vi "数据处理整合 (子VI).vi"(11 "枚举":enum16{"实时数据排序", "小时数据排序"}(ring)) -> (3 "已排序的数组":string[](array[string]))   [LabVIEW 2016, in "数据传输系统-04.lvlib"]
uses:
  <userlib>/_OpenG.lib/array/array.llb/Remove Duplicates from 1D Array (String)__ogtk.vi
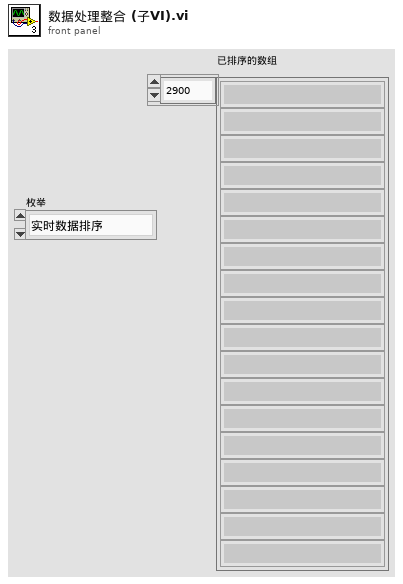
[diagram p1: front panel]
types:
  T1 = cluster{"PH":string[][], "CODCr":string[][], "氨氮":string[][], "CODMn":string[][], "总氮":string[][], "总磷":string[][], "电导率":string[][], "水温":string[][], "COD":string[][], "DO":string[][], "浊度":string[][], "叶绿素":string[][], "藻密度":string[][], "铜":string[][], "盐度":string[][], "水位":string[][], "流速":string[][], "方向":string[][], "瞬时流量":string[][], "累积流量":string[][], "正累积流量":string[][], "负累积流量":string[][], "亚硝酸盐":string[][], "硫化物":string[][], "ORP":string[][], "铅":string[][], "镉":string[][], "锌":string[][], "镍":string[][], "锰":string[][], "汞":string[][], "气温":string[][], "气压":string[][], "风速":string[][], "风向":string[][], "空气温度":string[][], "相对湿度":string[][], "分钟雨量":string[][], "小时雨量":string[][], "日雨量":string[][], "累积雨量":string[][], "盐度":string[][], "磷酸盐":string[][], "硝氮":string[][], "氟化物":string[][], "挥发酚":string[][], "氯化物":string[][], "蓝绿藻":string[][], "余氯":string[][], "综合生物毒性":string[][], "水深":string[][]}
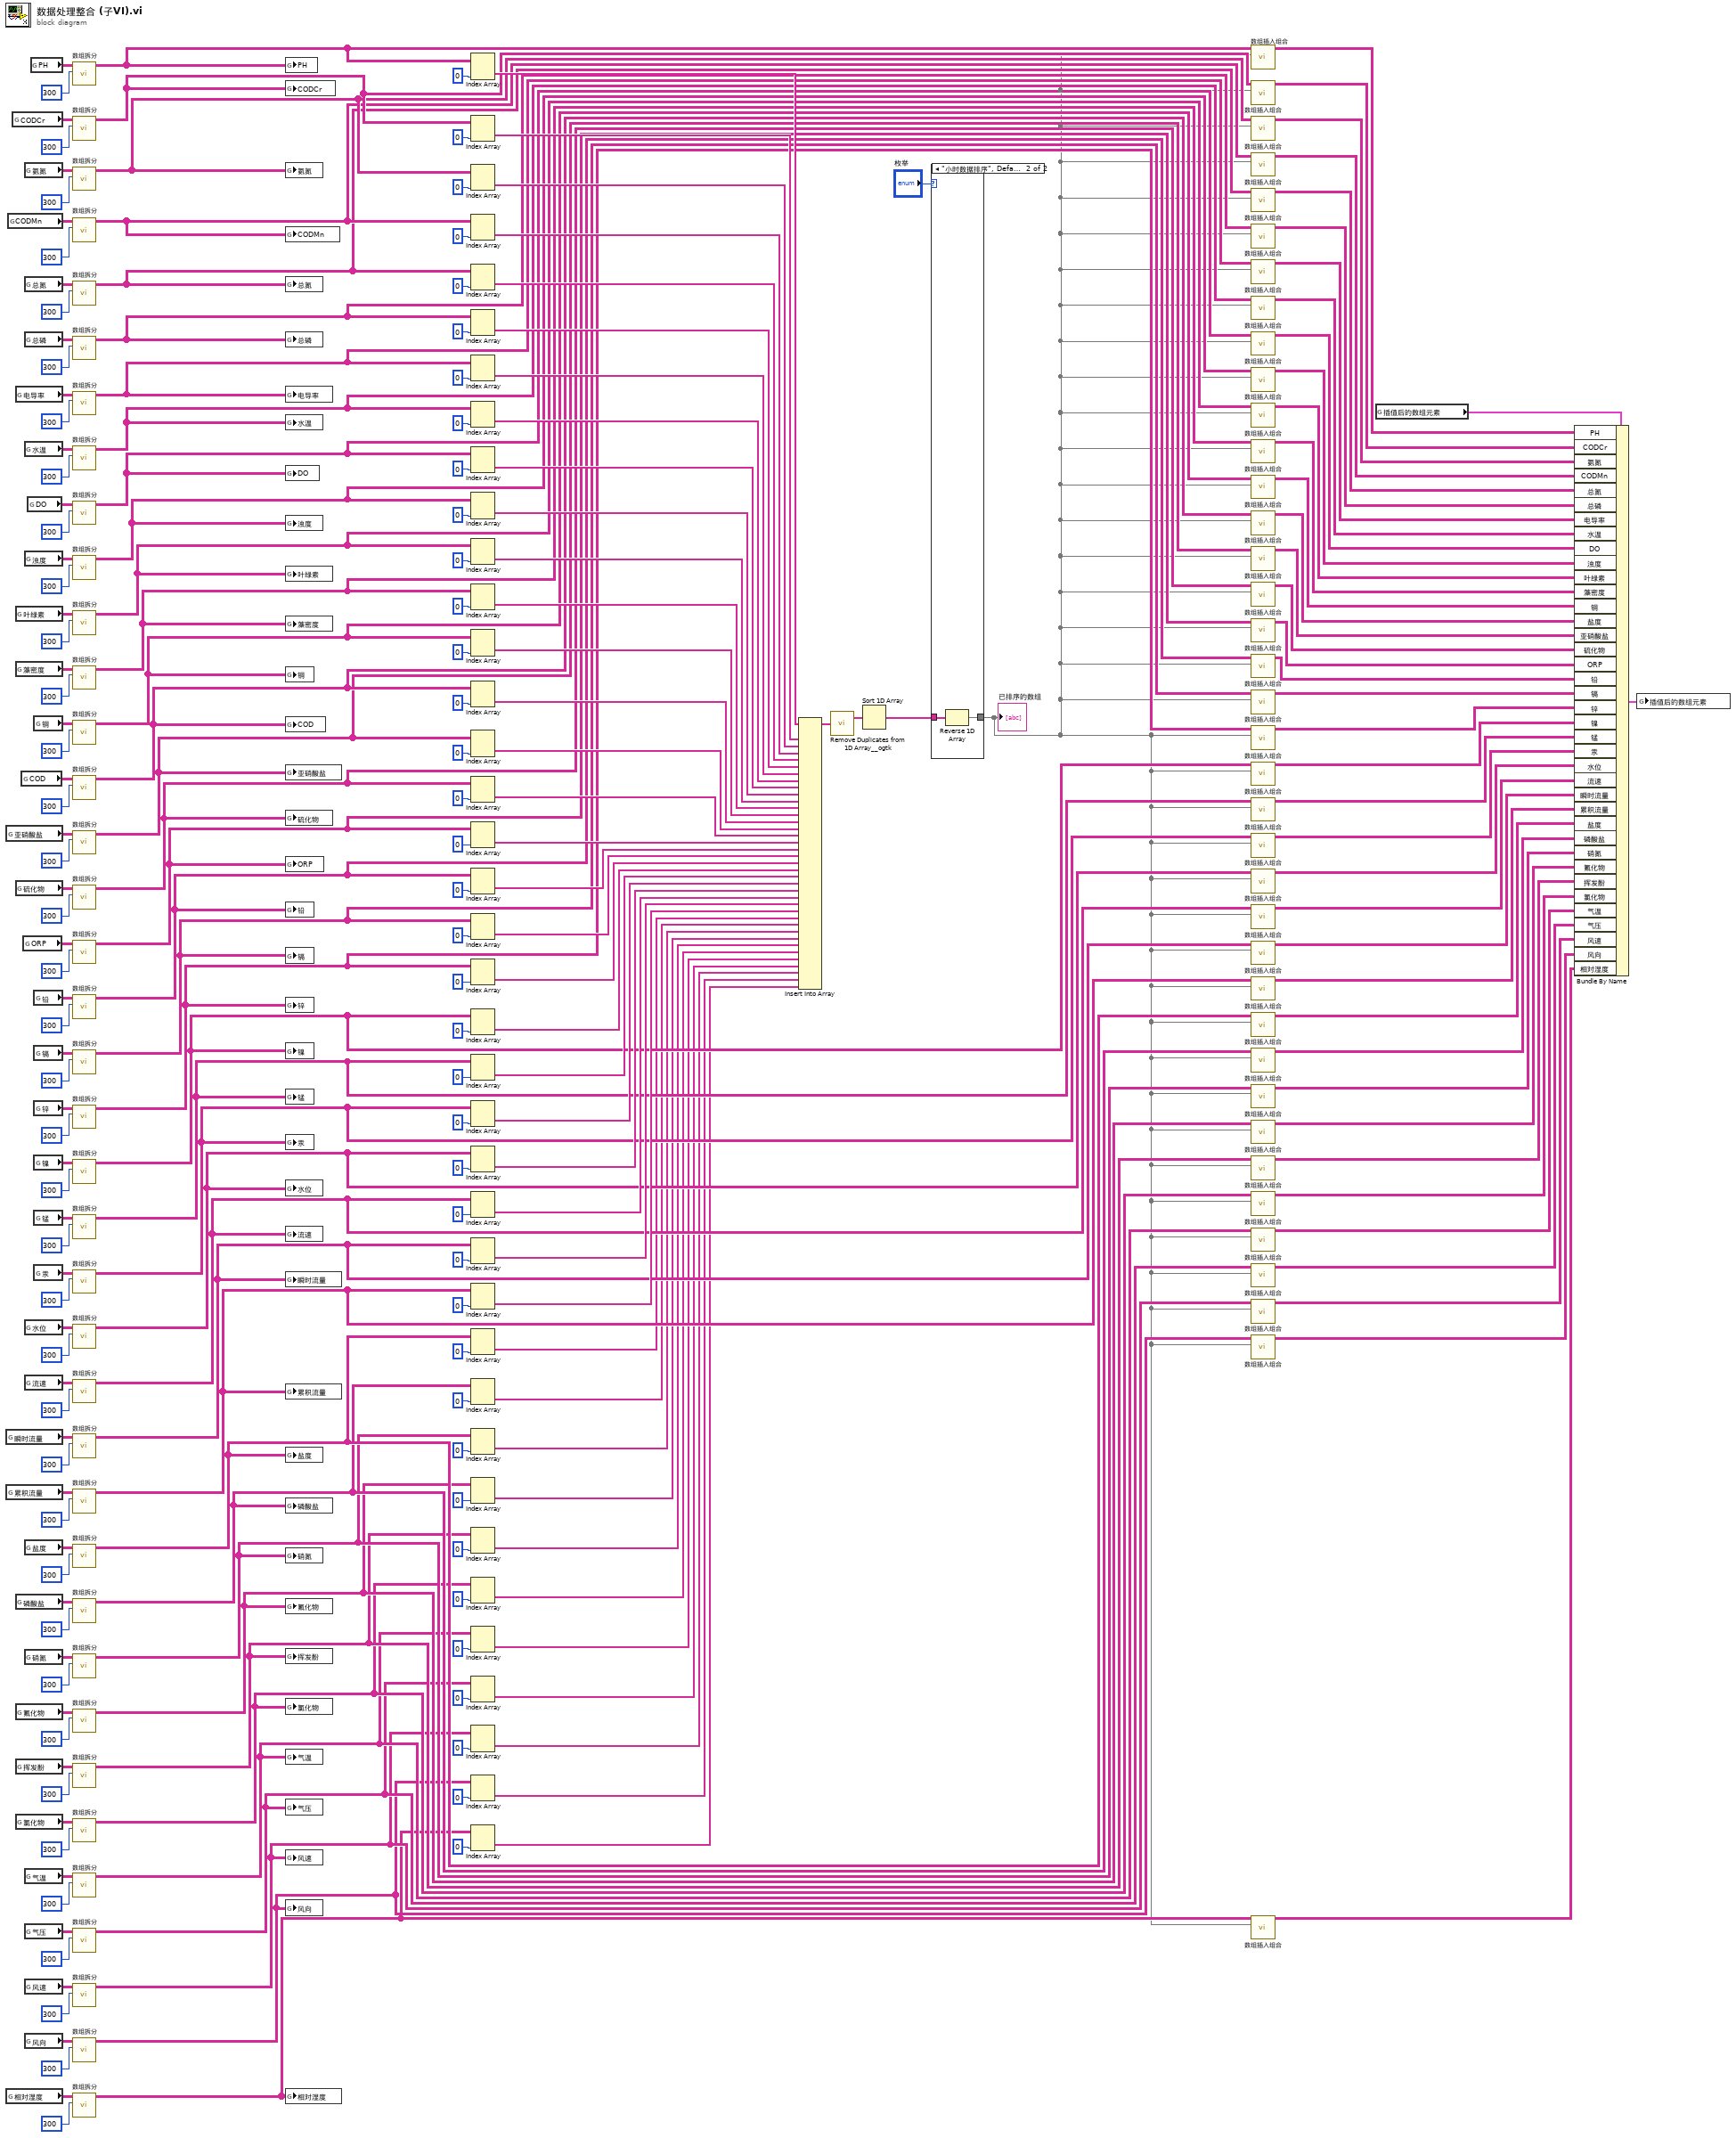
[diagram p0: block diagram]
diagram:
  n1 = global read "全局 所有参数.vi" "亚硝酸盐"() -> (w99:string[][])
  n2 = global read "全局 所有参数.vi" "瞬时流量"() -> (w75:string[][])
  n3 = global read "全局 所有参数.vi" "累积流量"() -> (w74:string[][])
  n4 = global read "全局 所有参数.vi" "相对湿度"() -> (w20:string[][])
  n5 = global read "全局 所有参数.vi" "CODMn"() -> (w138:string[][])
  n6 = global read "全局 所有参数.vi" "CODCr"() -> (w144:string[][])
  n7 = global read "全局 所有参数.vi" "电导率"() -> (w128:string[][])
  n8 = global read "全局 所有参数.vi" "叶绿素"() -> (w115:string[][])
  n9 = global read "全局 所有参数.vi" "藻密度"() -> (w114:string[][])
  n10 = global read "全局 所有参数.vi" "硫化物"() -> (w98:string[][])
  n11 = global read "全局 所有参数.vi" "磷酸盐"() -> (w60:string[][])
  n12 = global read "全局 所有参数.vi" "氟化物"() -> (w49:string[][])
  n13 = global read "全局 所有参数.vi" "挥发酚"() -> (w44:string[][])
  n14 = global read "全局 所有参数.vi" "氯化物"() -> (w43:string[][])
  n15 = global read "全局 所有参数.vi" "COD"() -> (w112:string[][])
  n16 = global read "全局 所有参数.vi" "ORP"() -> (w97:string[][])
  n17 = global read "全局 所有参数.vi" "氨氮"() -> (w141:string[][])
  n18 = global read "全局 所有参数.vi" "总氮"() -> (w135:string[][])
  n19 = global read "全局 所有参数.vi" "总磷"() -> (w129:string[][])
  n20 = global read "全局 所有参数.vi" "水温"() -> (w127:string[][])
  n21 = global read "全局 所有参数.vi" "浊度"() -> (w116:string[][])
  n22 = global read "全局 所有参数.vi" "水位"() -> (w77:string[][])
  n23 = global read "全局 所有参数.vi" "流速"() -> (w76:string[][])
  n24 = global read "全局 所有参数.vi" "盐度"() -> (w61:string[][])
  n25 = global read "全局 所有参数.vi" "硝氮"() -> (w59:string[][])
  n26 = global read "全局 所有参数.vi" "气温"() -> (w29:string[][])
  n27 = global read "全局 所有参数.vi" "气压"() -> (w30:string[][])
  n28 = global read "全局 所有参数.vi" "风速"() -> (w24:string[][])
  n29 = global read "全局 所有参数.vi" "风向"() -> (w23:string[][])
  n30 = global read "全局 所有参数.vi" "DO"() -> (w126:string[][])
  n31 = global read "全局 所有参数.vi" "PH"() -> (w147:string[][])
  n32 = global read "全局 所有参数.vi" "铜"() -> (w113:string[][])
  n33 = global read "全局 所有参数.vi" "铅"() -> (w96:string[][])
  n34 = global read "全局 所有参数.vi" "镉"() -> (w95:string[][])
  n35 = global read "全局 所有参数.vi" "锌"() -> (w94:string[][])
  n36 = global read "全局 所有参数.vi" "镍"() -> (w93:string[][])
  n37 = global read "全局 所有参数.vi" "锰"() -> (w79:string[][])
  n38 = global read "全局 所有参数.vi" "汞"() -> (w78:string[][])
  n39 = call "数组拆分.vi"("拆分大小"=300, "输入数据"=w147) -> ("输出数组"=w146:string[][])  [unwired: 8 in, 1 out]
  n40 = call "数组拆分.vi"("拆分大小"=300, "输入数据"=w144) -> ("输出数组"=w143:string[][])  [unwired: 8 in, 1 out]
  n41 = call "数组拆分.vi"("拆分大小"=300, "输入数据"=w141) -> ("输出数组"=w140:string[][])  [unwired: 8 in, 1 out]
  n42 = call "数组拆分.vi"("拆分大小"=300, "输入数据"=w138) -> ("输出数组"=w137:string[][])  [unwired: 8 in, 1 out]
  n43 = call "数组拆分.vi"("拆分大小"=300, "输入数据"=w135) -> ("输出数组"=w134:string[][])  [unwired: 8 in, 1 out]
  n44 = call "数组拆分.vi"("拆分大小"=300, "输入数据"=w129) -> ("输出数组"=w122:string[][])  [unwired: 8 in, 1 out]
  n45 = call "数组拆分.vi"("拆分大小"=300, "输入数据"=w128) -> ("输出数组"=w123:string[][])  [unwired: 8 in, 1 out]
  n46 = call "数组拆分.vi"("拆分大小"=300, "输入数据"=w127) -> ("输出数组"=w124:string[][])  [unwired: 8 in, 1 out]
  n47 = call "数组拆分.vi"("拆分大小"=300, "输入数据"=w126) -> ("输出数组"=w125:string[][])  [unwired: 8 in, 1 out]
  n48 = call "数组拆分.vi"("拆分大小"=300, "输入数据"=w116) -> ("输出数组"=w111:string[][])  [unwired: 8 in, 1 out]
  n49 = call "数组拆分.vi"("拆分大小"=300, "输入数据"=w115) -> ("输出数组"=w107:string[][])  [unwired: 8 in, 1 out]
  n50 = call "数组拆分.vi"("拆分大小"=300, "输入数据"=w114) -> ("输出数组"=w108:string[][])  [unwired: 8 in, 1 out]
  n51 = call "数组拆分.vi"("拆分大小"=300, "输入数据"=w113) -> ("输出数组"=w109:string[][])  [unwired: 8 in, 1 out]
  n52 = call "数组拆分.vi"("拆分大小"=300, "输入数据"=w112) -> ("输出数组"=w110:string[][])  [unwired: 8 in, 1 out]
  n53 = call "数组拆分.vi"("拆分大小"=300, "输入数据"=w99) -> ("输出数组"=w92:string[][])  [unwired: 8 in, 1 out]
  n54 = call "数组拆分.vi"("拆分大小"=300, "输入数据"=w98) -> ("输出数组"=w91:string[][])  [unwired: 8 in, 1 out]
  n55 = call "数组拆分.vi"("拆分大小"=300, "输入数据"=w97) -> ("输出数组"=w90:string[][])  [unwired: 8 in, 1 out]
  n56 = call "数组拆分.vi"("拆分大小"=300, "输入数据"=w96) -> ("输出数组"=w89:string[][])  [unwired: 8 in, 1 out]
  n57 = call "数组拆分.vi"("拆分大小"=300, "输入数据"=w95) -> ("输出数组"=w88:string[][])  [unwired: 8 in, 1 out]
  n58 = call "数组拆分.vi"("拆分大小"=300, "输入数据"=w94) -> ("输出数组"=w87:string[][])  [unwired: 8 in, 1 out]
  n59 = call "数组拆分.vi"("拆分大小"=300, "输入数据"=w93) -> ("输出数组"=w86:string[][])  [unwired: 8 in, 1 out]
  n60 = call "数组拆分.vi"("拆分大小"=300, "输入数据"=w79) -> ("输出数组"=w73:string[][])  [unwired: 8 in, 1 out]
  n61 = call "数组拆分.vi"("拆分大小"=300, "输入数据"=w78) -> ("输出数组"=w71:string[][])  [unwired: 8 in, 1 out]
  n62 = call "数组拆分.vi"("拆分大小"=300, "输入数据"=w77) -> ("输出数组"=w72:string[][])  [unwired: 8 in, 1 out]
  n63 = call "数组拆分.vi"("拆分大小"=300, "输入数据"=w76) -> ("输出数组"=w70:string[][])  [unwired: 8 in, 1 out]
  n64 = call "数组拆分.vi"("拆分大小"=300, "输入数据"=w75) -> ("输出数组"=w69:string[][])  [unwired: 8 in, 1 out]
  n65 = call "数组拆分.vi"("拆分大小"=300, "输入数据"=w74) -> ("输出数组"=w68:string[][])  [unwired: 8 in, 1 out]
  n66 = call "数组拆分.vi"("拆分大小"=300, "输入数据"=w61) -> ("输出数组"=w55:string[][])  [unwired: 8 in, 1 out]
  n67 = call "数组拆分.vi"("拆分大小"=300, "输入数据"=w60) -> ("输出数组"=w54:string[][])  [unwired: 8 in, 1 out]
  n68 = call "数组拆分.vi"("拆分大小"=300, "输入数据"=w59) -> ("输出数组"=w53:string[][])  [unwired: 8 in, 1 out]
  n69 = call "数组拆分.vi"("拆分大小"=300, "输入数据"=w49) -> ("输出数组"=w39:string[][])  [unwired: 8 in, 1 out]
  n70 = call "数组拆分.vi"("拆分大小"=300, "输入数据"=w44) -> ("输出数组"=w36:string[][])  [unwired: 8 in, 1 out]
  n71 = call "数组拆分.vi"("拆分大小"=300, "输入数据"=w43) -> ("输出数组"=w35:string[][])  [unwired: 8 in, 1 out]
  n72 = call "数组拆分.vi"("拆分大小"=300, "输入数据"=w29) -> ("输出数组"=w12:string[][])  [unwired: 8 in, 1 out]
  n73 = call "数组拆分.vi"("拆分大小"=300, "输入数据"=w30) -> ("输出数组"=w11:string[][])  [unwired: 8 in, 1 out]
  n74 = call "数组拆分.vi"("拆分大小"=300, "输入数据"=w24) -> ("输出数组"=w10:string[][])  [unwired: 8 in, 1 out]
  n75 = call "数组拆分.vi"("拆分大小"=300, "输入数据"=w23) -> ("输出数组"=w9:string[][])  [unwired: 8 in, 1 out]
  n76 = call "数组拆分.vi"("拆分大小"=300, "输入数据"=w20) -> ("输出数组"=w8:string[][])  [unwired: 8 in, 1 out]
  n77 = global write "全局 所有参数.vi" "PH"(w146) -> ()
  n78 = global write "全局 所有参数.vi" "CODCr"(w143) -> ()
  n79 = global write "全局 所有参数.vi" "氨氮"(w140) -> ()
  n80 = global write "全局 所有参数.vi" "CODMn"(w137) -> ()
  n81 = global write "全局 所有参数.vi" "总氮"(w134) -> ()
  n82 = global write "全局 所有参数.vi" "总磷"(w122) -> ()
  n83 = global write "全局 所有参数.vi" "电导率"(w123) -> ()
  n84 = global write "全局 所有参数.vi" "水温"(w124) -> ()
  n85 = global write "全局 所有参数.vi" "DO"(w125) -> ()
  n86 = global write "全局 所有参数.vi" "浊度"(w111) -> ()
  n87 = global write "全局 所有参数.vi" "叶绿素"(w107) -> ()
  n88 = global write "全局 所有参数.vi" "藻密度"(w108) -> ()
  n89 = global write "全局 所有参数.vi" "铜"(w109) -> ()
  n90 = global write "全局 所有参数.vi" "COD"(w110) -> ()
  n91 = global write "全局 所有参数.vi" "亚硝酸盐"(w92) -> ()
  n92 = global write "全局 所有参数.vi" "硫化物"(w91) -> ()
  n93 = global write "全局 所有参数.vi" "ORP"(w90) -> ()
  n94 = global write "全局 所有参数.vi" "铅"(w89) -> ()
  n95 = global write "全局 所有参数.vi" "镉"(w88) -> ()
  n96 = global write "全局 所有参数.vi" "锌"(w87) -> ()
  n97 = global write "全局 所有参数.vi" "镍"(w86) -> ()
  n98 = global write "全局 所有参数.vi" "锰"(w73) -> ()
  n99 = global write "全局 所有参数.vi" "汞"(w71) -> ()
  n100 = global write "全局 所有参数.vi" "水位"(w72) -> ()
  n101 = global write "全局 所有参数.vi" "流速"(w70) -> ()
  n102 = global write "全局 所有参数.vi" "瞬时流量"(w69) -> ()
  n103 = global write "全局 所有参数.vi" "累积流量"(w68) -> ()
  n104 = global write "全局 所有参数.vi" "盐度"(w55) -> ()
  n105 = global write "全局 所有参数.vi" "磷酸盐"(w54) -> ()
  n106 = global write "全局 所有参数.vi" "硝氮"(w53) -> ()
  n107 = global write "全局 所有参数.vi" "氟化物"(w39) -> ()
  n108 = global write "全局 所有参数.vi" "挥发酚"(w36) -> ()
  n109 = global write "全局 所有参数.vi" "氯化物"(w35) -> ()
  n110 = global write "全局 所有参数.vi" "气温"(w12) -> ()
  n111 = global write "全局 所有参数.vi" "气压"(w11) -> ()
  n112 = global write "全局 所有参数.vi" "风速"(w10) -> ()
  n113 = global write "全局 所有参数.vi" "风向"(w9) -> ()
  n114 = global write "全局 所有参数.vi" "相对湿度"(w8) -> ()
  n115 = Index Array(array=w146, index (col)=0 ("索引 (行)")) -> (element=w211:string[])  [unwired: 1 in]
  n116 = Index Array(array=w143, index (col)=0 ("索引 (行)")) -> (element=w212:string[])  [unwired: 1 in]
  n117 = Index Array(array=w140, index (col)=0 ("索引 (行)")) -> (element=w213:string[])  [unwired: 1 in]
  n118 = Index Array(array=w137, index (col)=0 ("索引 (行)")) -> (element=w214:string[])  [unwired: 1 in]
  n119 = Index Array(array=w134, index (col)=0 ("索引 (行)")) -> (element=w215:string[])  [unwired: 1 in]
  n120 = Index Array(array=w122, index (col)=0 ("索引 (行)")) -> (element=w216:string[])  [unwired: 1 in]
  n121 = Index Array(array=w123, index (col)=0 ("索引 (行)")) -> (element=w217:string[])  [unwired: 1 in]
  n122 = Index Array(array=w124, index (col)=0 ("索引 (行)")) -> (element=w218:string[])  [unwired: 1 in]
  n123 = Index Array(array=w125, index (col)=0 ("索引 (行)")) -> (element=w219:string[])  [unwired: 1 in]
  n124 = Index Array(array=w111, index (col)=0 ("索引 (行)")) -> (element=w220:string[])  [unwired: 1 in]
  n125 = Index Array(array=w107, index (col)=0 ("索引 (行)")) -> (element=w221:string[])  [unwired: 1 in]
  n126 = Index Array(array=w108, index (col)=0 ("索引 (行)")) -> (element=w222:string[])  [unwired: 1 in]
  n127 = Index Array(array=w109, index (col)=0 ("索引 (行)")) -> (element=w195:string[])  [unwired: 1 in]
  n128 = Index Array(array=w110, index (col)=0 ("索引 (行)")) -> (element=w194:string[])  [unwired: 1 in]
  n129 = Index Array(array=w92, index (col)=0 ("索引 (行)")) -> (element=w180:string[])  [unwired: 1 in]
  n130 = Index Array(array=w91, index (col)=0 ("索引 (行)")) -> (element=w181:string[])  [unwired: 1 in]
  n131 = Index Array(array=w90, index (col)=0 ("索引 (行)")) -> (element=w182:string[])  [unwired: 1 in]
  n132 = Index Array(array=w89, index (col)=0 ("索引 (行)")) -> (element=w172:string[])  [unwired: 1 in]
  n133 = Index Array(array=w88, index (col)=0 ("索引 (行)")) -> (element=w171:string[])  [unwired: 1 in]
  n134 = Index Array(array=w87, index (col)=0 ("索引 (行)")) -> (element=w170:string[])  [unwired: 1 in]
  n135 = Index Array(array=w86, index (col)=0 ("索引 (行)")) -> (element=w166:string[])  [unwired: 1 in]
  n136 = Index Array(array=w73, index (col)=0 ("索引 (行)")) -> (element=w165:string[])  [unwired: 1 in]
  n137 = Index Array(array=w71, index (col)=0 ("索引 (行)")) -> (element=w164:string[])  [unwired: 1 in]
  n138 = Index Array(array=w72, index (col)=0 ("索引 (行)")) -> (element=w156:string[])  [unwired: 1 in]
  n139 = Index Array(array=w70, index (col)=0 ("索引 (行)")) -> (element=w155:string[])  [unwired: 1 in]
  n140 = Index Array(array=w69, index (col)=0 ("索引 (行)")) -> (element=w154:string[])  [unwired: 1 in]
  n141 = Index Array(array=w68, index (col)=0 ("索引 (行)")) -> (element=w153:string[])  [unwired: 1 in]
  n142 = Index Array(array=w55, index (col)=0 ("索引 (行)")) -> (element=w58:string[])  [unwired: 1 in]
  n143 = Index Array(array=w54, index (col)=0 ("索引 (行)")) -> (element=w57:string[])  [unwired: 1 in]
  n144 = Index Array(array=w53, index (col)=0 ("索引 (行)")) -> (element=w56:string[])  [unwired: 1 in]
  n145 = Index Array(array=w39, index (col)=0 ("索引 (行)")) -> (element=w40:string[])  [unwired: 1 in]
  n146 = Index Array(array=w36, index (col)=0 ("索引 (行)")) -> (element=w38:string[])  [unwired: 1 in]
  n147 = Index Array(array=w35, index (col)=0 ("索引 (行)")) -> (element=w37:string[])  [unwired: 1 in]
  n148 = Index Array(array=w12, index (col)=0 ("索引 (行)")) -> (element=w17:string[])  [unwired: 1 in]
  n149 = Index Array(array=w11, index (col)=0 ("索引 (行)")) -> (element=w16:string[])  [unwired: 1 in]
  n150 = Index Array(array=w10, index (col)=0 ("索引 (行)")) -> (element=w15:string[])  [unwired: 1 in]
  n151 = Index Array(array=w9, index (col)=0 ("索引 (行)")) -> (element=w14:string[])  [unwired: 1 in]
  n152 = Index Array(array=w8, index (col)=0 ("索引 (行)")) -> (element=w13:string[])  [unwired: 1 in]
  n153 = Insert Into Array(array=w211, new element #1=w212, new element #2=w213, new element #3=w214, new element #4=w215, new element #5=w216, new element #6=w217, new element #7=w218, new element #8=w219, new element #9=w220, new element #10=w221, new element #11=w222, new element #12=w195, new element #13=w194, new element #14=w180, new element #15=w181, new element #16=w182, new element #17=w172, new element #18=w171, new element #19=w170, new element #20=w166, new element #21=w165, new element #22=w164, new element #23=w156, new element #24=w155, new element #25=w154, new element #26=w153, new element #27=w58, new element #28=w57, new element #29=w56, new element #30=w40, new element #31=w38, new element #32=w37, new element #33=w17, new element #34=w16, new element #35=w15, new element #36=w14, new element #37=w13) -> (w223:string[])  [unwired: 1 in]
  n154 = call-poly <userlib>:"Remove Duplicates from 1D Array__ogtk.vi"("Input Array"=w223) -> ("Output Array"=w210:string[])  [unwired: 1 out]
  n155 = Sort 1D Array(array=w210) -> (sorted array=w196:string[])
  n156 = case shown="\"小时数据排序\", Default" "枚举" {
    tunnel: w196 -> [w236 w238]
    tunnel: [w236 w237] -> w2
    frame "实时数据排序" {
    }
    frame "小时数据排序", Default {
      n157 = Reverse 1D Array(array=w238) -> (reversed array=w237:string[])
    }
  }
  "已排序的数组" <- w2
  n158 = call "数组插入组合.vi"("排序后的一维数组"=w2, "输入数组"=w146) -> ("输出结果"=w224:string[][])  [unwired: 9 in]
  n159 = call "数组插入组合.vi"("排序后的一维数组"=w2, "输入数组"=w143) -> ("输出结果"=w225:string[][])  [unwired: 9 in]
  n160 = call "数组插入组合.vi"("排序后的一维数组"=w2, "输入数组"=w140) -> ("输出结果"=w226:string[][])  [unwired: 9 in]
  n161 = call "数组插入组合.vi"("排序后的一维数组"=w2, "输入数组"=w137) -> ("输出结果"=w227:string[][])  [unwired: 9 in]
  n162 = call "数组插入组合.vi"("排序后的一维数组"=w2, "输入数组"=w134) -> ("输出结果"=w228:string[][])  [unwired: 9 in]
  n163 = call "数组插入组合.vi"("排序后的一维数组"=w2, "输入数组"=w122) -> ("输出结果"=w229:string[][])  [unwired: 9 in]
  n164 = call "数组插入组合.vi"("排序后的一维数组"=w2, "输入数组"=w123) -> ("输出结果"=w230:string[][])  [unwired: 9 in]
  n165 = call "数组插入组合.vi"("排序后的一维数组"=w2, "输入数组"=w124) -> ("输出结果"=w231:string[][])  [unwired: 9 in]
  n166 = call "数组插入组合.vi"("排序后的一维数组"=w2, "输入数组"=w125) -> ("输出结果"=w232:string[][])  [unwired: 9 in]
  n167 = call "数组插入组合.vi"("排序后的一维数组"=w2, "输入数组"=w111) -> ("输出结果"=w233:string[][])  [unwired: 9 in]
  n168 = call "数组插入组合.vi"("排序后的一维数组"=w2, "输入数组"=w107) -> ("输出结果"=w234:string[][])  [unwired: 9 in]
  n169 = call "数组插入组合.vi"("排序后的一维数组"=w2, "输入数组"=w108) -> ("输出结果"=w235:string[][])  [unwired: 9 in]
  n170 = call "数组插入组合.vi"("排序后的一维数组"=w2, "输入数组"=w109) -> ("输出结果"=w193:string[][])  [unwired: 9 in]
  n171 = call "数组插入组合.vi"("排序后的一维数组"=w2, "输入数组"=w110) -> ("输出结果"=w192:string[][])  [unwired: 9 in]
  n172 = call "数组插入组合.vi"("排序后的一维数组"=w2, "输入数组"=w92) -> ("输出结果"=w185:string[][])  [unwired: 9 in]
  n173 = call "数组插入组合.vi"("排序后的一维数组"=w2, "输入数组"=w91) -> ("输出结果"=w183:string[][])  [unwired: 9 in]
  n174 = call "数组插入组合.vi"("排序后的一维数组"=w2, "输入数组"=w90) -> ("输出结果"=w184:string[][])  [unwired: 9 in]
  n175 = call "数组插入组合.vi"("排序后的一维数组"=w2, "输入数组"=w89) -> ("输出结果"=w175:string[][])  [unwired: 9 in]
  n176 = call "数组插入组合.vi"("排序后的一维数组"=w2, "输入数组"=w88) -> ("输出结果"=w174:string[][])  [unwired: 9 in]
  n177 = call "数组插入组合.vi"("排序后的一维数组"=w2, "输入数组"=w87) -> ("输出结果"=w173:string[][])  [unwired: 9 in]
  n178 = call "数组插入组合.vi"("排序后的一维数组"=w2, "输入数组"=w86) -> ("输出结果"=w163:string[][])  [unwired: 9 in]
  n179 = call "数组插入组合.vi"("排序后的一维数组"=w2, "输入数组"=w73) -> ("输出结果"=w162:string[][])  [unwired: 9 in]
  n180 = call "数组插入组合.vi"("排序后的一维数组"=w2, "输入数组"=w71) -> ("输出结果"=w161:string[][])  [unwired: 9 in]
  n181 = call "数组插入组合.vi"("排序后的一维数组"=w2, "输入数组"=w72) -> ("输出结果"=w152:string[][])  [unwired: 9 in]
  n182 = call "数组插入组合.vi"("排序后的一维数组"=w2, "输入数组"=w70) -> ("输出结果"=w151:string[][])  [unwired: 9 in]
  n183 = call "数组插入组合.vi"("排序后的一维数组"=w2, "输入数组"=w69) -> ("输出结果"=w150:string[][])  [unwired: 9 in]
  n184 = call "数组插入组合.vi"("排序后的一维数组"=w2, "输入数组"=w68) -> ("输出结果"=w149:string[][])  [unwired: 9 in]
  n185 = call "数组插入组合.vi"("排序后的一维数组"=w2, "输入数组"=w55) -> ("输出结果"=w52:string[][])  [unwired: 9 in]
  n186 = call "数组插入组合.vi"("排序后的一维数组"=w2, "输入数组"=w54) -> ("输出结果"=w51:string[][])  [unwired: 9 in]
  n187 = call "数组插入组合.vi"("排序后的一维数组"=w2, "输入数组"=w53) -> ("输出结果"=w50:string[][])  [unwired: 9 in]
  n188 = call "数组插入组合.vi"("排序后的一维数组"=w2, "输入数组"=w39) -> ("输出结果"=w34:string[][])  [unwired: 9 in]
  n189 = call "数组插入组合.vi"("排序后的一维数组"=w2, "输入数组"=w36) -> ("输出结果"=w33:string[][])  [unwired: 9 in]
  n190 = call "数组插入组合.vi"("排序后的一维数组"=w2, "输入数组"=w35) -> ("输出结果"=w1:string[][])  [unwired: 9 in]
  n191 = call "数组插入组合.vi"("排序后的一维数组"=w2, "输入数组"=w12) -> ("输出结果"=w7:string[][])  [unwired: 9 in]
  n192 = call "数组插入组合.vi"("排序后的一维数组"=w2, "输入数组"=w11) -> ("输出结果"=w6:string[][])  [unwired: 9 in]
  n193 = call "数组插入组合.vi"("排序后的一维数组"=w2, "输入数组"=w10) -> ("输出结果"=w5:string[][])  [unwired: 9 in]
  n194 = call "数组插入组合.vi"("排序后的一维数组"=w2, "输入数组"=w9) -> ("输出结果"=w4:string[][])  [unwired: 9 in]
  n195 = call "数组插入组合.vi"("排序后的一维数组"=w2, "输入数组"=w8) -> ("输出结果"=w3:string[][])  [unwired: 9 in]
  n196 = global read "插值后的新数组.vi" "插值后的数组元素"() -> (w189:T1)
  n197 = Bundle By Name(cluster=w189, "PH"=w224, "CODCr"=w225, "氨氮"=w226, "CODMn"=w227, "总氮"=w228, "总磷"=w229, "电导率"=w230, "水温"=w231, "DO"=w232, "浊度"=w233, "叶绿素"=w234, "藻密度"=w235, "铜"=w193, "盐度"=w192, "亚硝酸盐"=w185, "硫化物"=w183, "ORP"=w184, "铅"=w175, "镉"=w174, "锌"=w173, "镍"=w163, "锰"=w162, "汞"=w161, "水位"=w152, "流速"=w151, "瞬时流量"=w150, "累积流量"=w149, "盐度"=w52, "磷酸盐"=w51, "硝氮"=w50, "氟化物"=w34, "挥发酚"=w33, "氯化物"=w1, "气温"=w7, "气压"=w6, "风速"=w5, "风向"=w4, "相对湿度"=w3) -> (w179:T1)
  n198 = global write "插值后的新数组.vi" "插值后的数组元素"(w179) -> ()
